vi "truncate_actual_array.vi"() -> ()   [LabVIEW 2014, in "double_array.lvclass"]
uses:
  double_array.lvclass
  double_array.lvclass/double_array.ctl
panel:
  out "output_double_array.lvclass":refnum<class "double_array.lvclass">
  out "truncated_array":dbl[](array[numeric])
  in  "input_double_array.lvclass":refnum<class "double_array.lvclass">
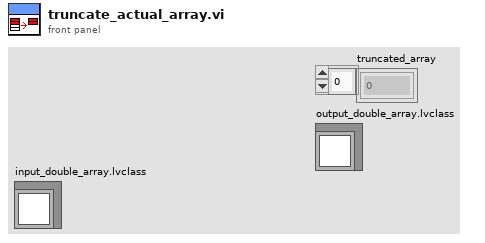
[diagram p1: front panel]
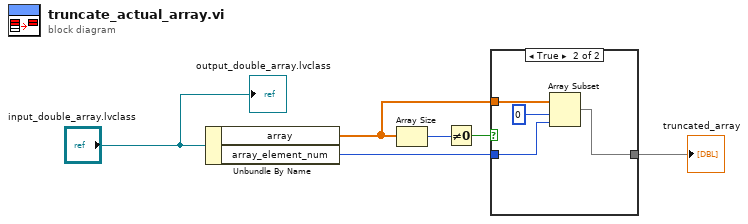
[diagram p0: block diagram]
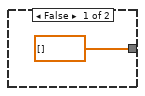
[diagram p2: hidden frame]
diagram:
  n1 = Unbundle By Name("input_double_array.lvclass") -> ("array"=w1:dbl[], "array_element_num"=w3:u32)
  n2 = Array Size(array=w1) -> (size(s)=w5:i32)
  n3 = Not Equal To 0?(x=w5) -> (x != 0?=w4:bool)
  n4 = case shown="True" w4 {
    tunnel: w3 -> [_ w9]
    tunnel: [dbl[] [] ("array") w8] -> w2
    tunnel: w1 -> [_ w11]
    frame False {
    }
    frame True {
      n5 = Array Subset(array=w11, index=0, length=w9) -> (w8:dbl[])
    }
  }
  "truncated_array" <- w2
  "output_double_array.lvclass" <- "input_double_array.lvclass"
